vi "Pulse Mode - Configure Start Angle.vi"(8 "error in (no error)":errorcluster, 10 "Start Angle(degree)":u16 max=359, 11 "VISA resource name":refnum<visa-resource-name>) -> (0 "error out":errorcluster, 3 "VISA resource name out":refnum<visa-resource-name>)   [LabVIEW 2014, in "Associated Power Technologies 8500 Series.lvlib"]
doc: "Configure the start angle.\n\n<B>Note:</B>\nRange : 0 ~ 359\n\nDefault value: 0"
uses:
  <instrlib>/Associated Power Technologies 8500 Series/Associated Power Technologies 8500 Series.lvlib
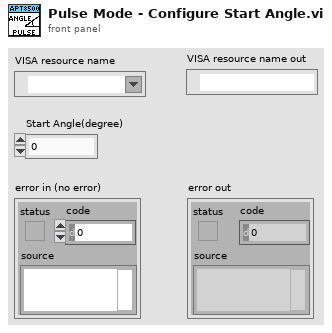
[diagram p1: front panel]
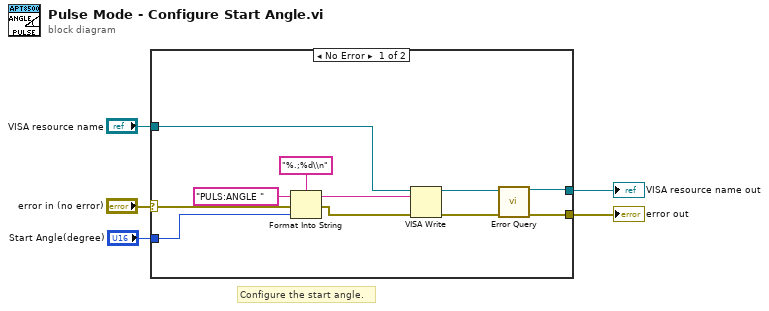
[diagram p0: block diagram]
diagram:
  # "Configure the start angle."
  n1 = case shown="No Error" "error in (no error)" {
    selector: "error in (no error)" -> [w15 w17]
    tunnel: "Start Angle(degree)" -> [w16 _]
    tunnel: "VISA resource name" -> [w11 w18]
    tunnel: [w8 w18] -> w2
    tunnel: [w6 w17] -> w1
    frame No Error {
      n2 = Format Into String(format string="%.;%d\\n", initial string="PULS:ANGLE " ("command"), error in=w15, w16) -> (resulting string=w10:string, error out=w14:errorcluster)
      n3 = VISA Write(VISA resource name=w11, write buffer=w10, error in (no error)=w14) -> (VISA resource name out=w9:refnum<visa-resource-name>, error out=w7:errorcluster)  [unwired: 1 out]
      n4 = call <instrlib>:"Error Query.vi"("VISA resource name"=w9, "error in (no error)"=w7) -> ("VISA resource name out"=w8:refnum<visa-resource-name>, "error out"=w6:errorcluster)  [unwired: 10 in, 2 out]
    }
    frame Error {
    }
  }
  "VISA resource name out" <- w2
  "error out" <- w1
